vi "BuildCall.vi"(7 "PythonConverter_BD in":refnum<class "PyConvBD.lvclass">, 8 "error in":errorcluster, 11 "Terminal in":refnum<class "Terminal.lvclass">) -> (0 "error out":errorcluster, 3 "Terminal out":refnum<class "Terminal.lvclass">, 5 "PythonConverter_BD out":refnum<class "PyConvBD.lvclass">)   [LabVIEW 2014, in "Raspberry Pi Compatible Compiler for LabVIEW.lvlib" / "Terminal.lvclass"]
uses:
  Terminal.lvclass
  Python/PythonConverter_BD/PyConvBD.lvclass
  Python/PythonConverter_BD/TypeDefs/NodeCall_TD.ctl
  Raspberry Pi Compatible Compiler for LabVIEW.lvlib
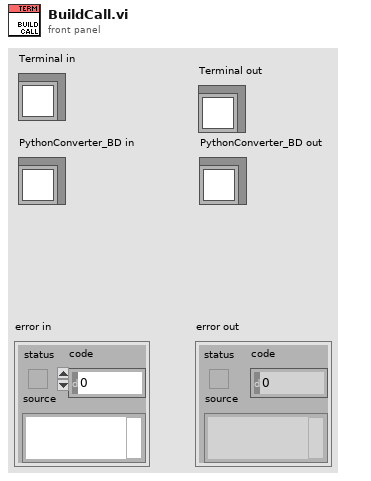
[diagram p1: front panel]
types:
  T1 = typedef "Raspberry Pi Compatible Compiler for LabVIEW.lvlib/NodeCall_TD.ctl" = cluster{"call":string, "collect":string, "Threaded":bool, "branches":string[]}
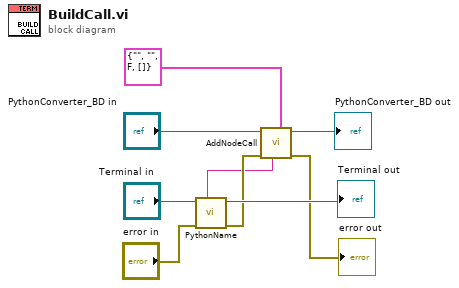
[diagram p0: block diagram]
diagram:
  n1 = call-dynamic "PythonName.vi"("error in"="error in", "Terminal in"="Terminal in") -> ("error out"=w4:errorcluster, "Terminal out"=→"Terminal out":refnum<class "Terminal.lvclass">, "UID"=w2:string)  [unwired: 6 in, 1 out]
  n2 = call "AddNodeCall.vi"("call"=T1 {"call"="", "collect"="", "Threaded"=FALSE, "branches"=[]}, "name"=w2, "error in"=w4, "PythonConverter_BD in"="PythonConverter_BD in") -> ("error out"=→"error out":errorcluster, "PythonConverter_BD out"=→"PythonConverter_BD out":refnum<class "PyConvBD.lvclass">)  [unwired: 4 in]
